vi "compare.vi"(10 "input variable 2":dbl, 11 "input variable":dbl) -> (1 "b":dbl, 2 "a":dbl, 3 "z":dbl, 4 "c":dbl)   [LabVIEW 2014]
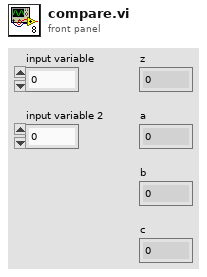
[diagram p1: front panel]
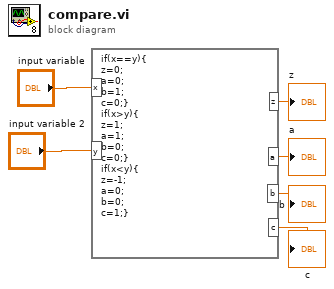
[diagram p0: block diagram]
diagram:
  n1 = formula code="if(x==y){\nz=0;\na=0;\nb=1;\nc=0;}\nif(x>y){\nz=1;\na=1;\nb=0;\nc=0;}\nif(x<y){\nz=-1;\na=0;\nb=0;\nc=1;}"("x"="input variable", "y"="input variable 2") -> ("z"=→"z":dbl, "a"=→"a":dbl, "b"=→"b":dbl, "c"=→"c":dbl)
